vi "Run.vi"(8 "error in (no error)":errorcluster, 11 "picoG in":refnum<class "picoG.lvclass">) -> (0 "error out":errorcluster, 3 "picoG out":refnum<class "picoG.lvclass">)   [LabVIEW 2020, in "PicoG-App.lvlib" / "picoG.lvclass"]
uses:
  picoG.lvclass
  picoG.lvclass/picoG.ctl
  App Watcher/App Watcher.lvclass
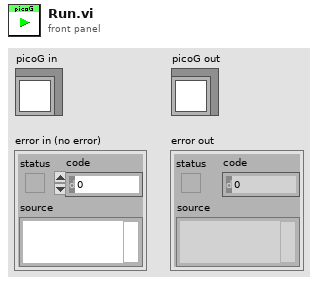
[diagram p1: front panel]
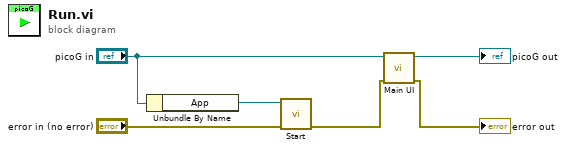
[diagram p0: block diagram]
diagram:
  n1 = Unbundle By Name("picoG in") -> ("App"=w3:refnum<class "App Watcher.lvclass">)
  n2 = call "Start.vi"("error in (no error)"="error in (no error)", "App Watcher in"=w3) -> ("error out"=w1:errorcluster)  [unwired: 8 in, 1 out]
  n3 = call "Main UI.vi"("error in (no error)"=w1, "picoG in"="picoG in") -> ("error out"=→"error out":errorcluster, "picoG out"=→"picoG out":refnum<class "picoG.lvclass">)  [unwired: 8 in]
